vi "LockinDAQ.Configure Sweep 4.vi"(8 "error in (no error)":errorcluster, 11 "LockinDAQ in":refnum<class "LockinDAQ.lvclass">) -> (0 "error out":errorcluster, 3 "LockinDAQ out":refnum<class "LockinDAQ.lvclass">)   [LabVIEW 2016, in "LockinDAQ.lvclass"]
uses:
  LockinDAQ.lvclass
  LockinDAQ.lvclass/LockinDAQ.ctl
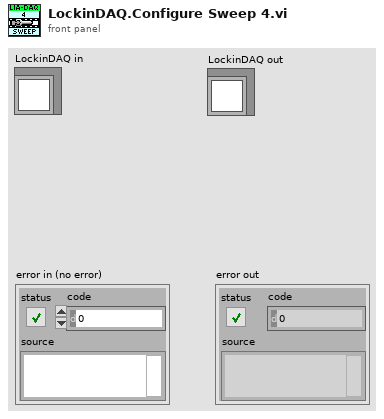
[diagram p1: front panel]
types:
  T1 = typedef "LockinDAQ.lvclass/AO-cluster.ctl" = cluster{"Ch":i32[], "Amp (V)":dbl[], "DC (V)":dbl[], "f (Hz)":dbl[], "Phase (°)":dbl[], "Function":T2[], "Sweep?":bool[]}
  T2 = typedef "LockinDAQ.lvclass/Function-enum.ctl" = enum16{"Sine", "Triangle", "Square", "Sawtooth"}
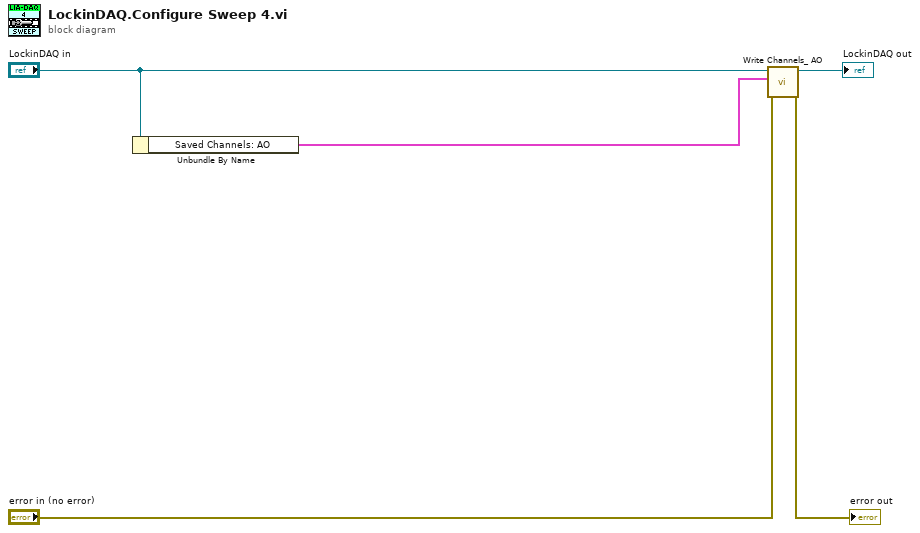
[diagram p0: block diagram]
diagram:
  n1 = Unbundle By Name("LockinDAQ in") -> ("Saved Channels: AO"=w1:T1)
  n2 = call "Write Channels_ AO.vi"("error in (no error)"="error in (no error)", "Channels: AO"=w1, "LockinDAQ"="LockinDAQ in") -> ("error out"=→"error out":errorcluster, "LockinDAQ out"=→"LockinDAQ out":refnum<class "LockinDAQ.lvclass">)  [unwired: 7 in]
